vi "Test API Creates Report Folder.vi"(8 "error in (no error)":errorcluster, 11 "API Test in":refnum<class "API Test.lvclass">) -> (0 "error out":errorcluster, 3 "API Test out":refnum<class "API Test.lvclass">)   [LabVIEW 2020, in "LUnit Tests.lvlib" / "API Test.lvclass"]
uses:
  API Test.lvclass
  source/Framework/Execution API/Execution API.lvclass
  <vilib>/Astemes/LUnit/Test Case.lvclass
  C:/Program Files (x86)/National Instruments/LabVIEW 2020/vi.lib/Astemes/LUnit/Test Case.lvclass
  Test Dummys/Test Test Case/Test Test Case.lvclass
panel:
  out "file or folder exists?":bool
  out "appended path":path
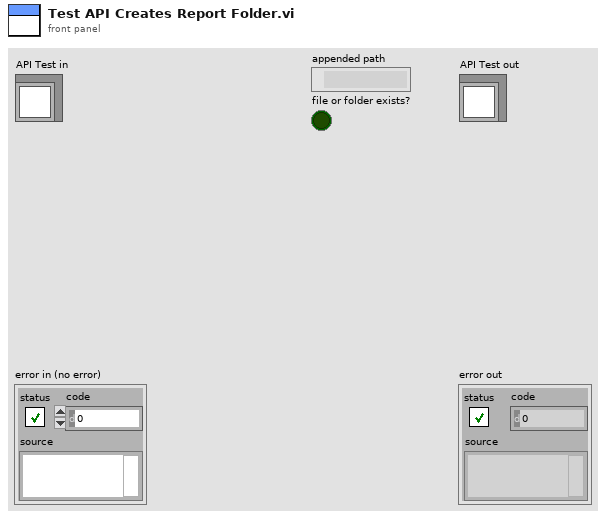
[diagram p1: front panel]
types:
  T1 = cluster{"Result Events":refnum<event-registration>, "Event Registration Refnum":refnum<event-registration>}
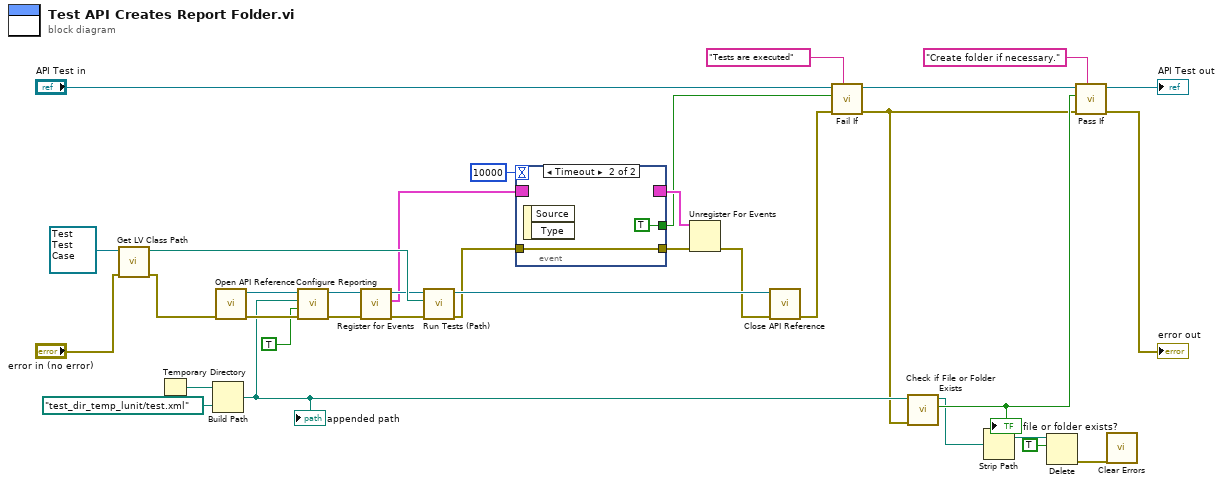
[diagram p0: block diagram]
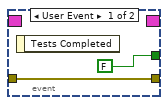
[diagram p2: hidden frame]
diagram:
  n1 = call <vilib>:"Get LV Class Path.vi"("error in (no error)"="error in (no error)", "object"=refnum<class "Test Test Case.lvclass"> refnum ("Test Test Case.lvclass")) -> ("error out"=w33:errorcluster, "class path"=w25:path)  [unwired: 8 in]
  n2 = Temporary Directory() -> (w24:path)
  n3 = Build Path(base path=w24, name or relative path=path "test_dir_temp_lunit/test.xml") -> (appended path=w21:path)
  "appended path" <- w21
  n4 = call "Open API Reference.vi"("error in (no error)"=w33) -> ("error out"=w27:errorcluster, "Execution API out"=w28:refnum<class "Execution API.lvclass">)  [unwired: 9 in]
  n5 = call "Configure Reporting.vi"("error in (no error)"=w27, "Autogenerate?"=TRUE, "Path"=w21, "Execution API In"=w28) -> ("error out"=w26:errorcluster, "Execution API Out"=w5:refnum<class "Execution API.lvclass">)  [unwired: 6 in]
  n6 = call "Register for Events.vi"("error in (no error)"=w26, "Execution API in"=w5) -> ("error out"=w6:errorcluster, "Event Registrations"=w3:T1, "Execution API out"=w4:refnum<class "Execution API.lvclass">)  [unwired: 7 in]
  n7 = call "Run Tests (Path).vi"("error in (no error)"=w6, "Project or Class Path"=w25, "Execution API In"=w4) -> ("error out"=w34:errorcluster, "Execution API Out"=w35:refnum<class "Execution API.lvclass">)  [unwired: 7 in]
  n8 = event shown="[1] Timeout" {
    selector: w3 -> [_ _]
    dyn-events: [_ _] -> w31
    timeout: 10000 -> [_ _]
    tunnel: [FALSE TRUE] -> w8
    tunnel: w34 -> [w36 w38]
    tunnel: [w36 w38] -> w30
    event User Event {
      n9 = event-data() -> ()  [unwired: 1 in, 1 out]
    }
    event Timeout {
      n10 = event-data() -> ()  [unwired: 1 in, 2 out]
    }
  }
  n11 = Unregister For Events(event registration refnum=w31, error in=w30) -> (error out=w32:errorcluster)
  n12 = call "Close API Reference.vi"("error in (no error)"=w32, "Execution API in"=w35) -> ("error out"=w13:errorcluster)  [unwired: 9 in]
  n13 = call <vilib>:"Fail If.vi"("Description"="Tests are executed", "error in (no error)"=w13, "Fail?"=w8, "LUnit Test Case In"="API Test in") -> ("error out"=w11:errorcluster, "LUnit Test Case Out"=w9:refnum<class "API Test.lvclass">)  [unwired: 6 in]
  n14 = call <vilib>:"Check if File or Folder Exists.vi"("error in (no error)"=w11, "path"=w21) -> ("file or folder exists?"=w18:bool, "dup path"=w17:path)  [unwired: 7 in, 1 out]
  "file or folder exists?" <- w18
  n15 = Strip Path(path=w17) -> (stripped path=w16:path)  [unwired: 1 out]
  n16 = Delete(path (use dialog)=w16, entire hierarchy (F)=TRUE) -> (error out=w1:errorcluster)  [unwired: 3 in, 2 out]
  n17 = call <vilib>:"Pass If.vi"("Description"="Create folder if necessary.", "error in (no error)"=w11, "Pass?"=w18, "LUnit Test Case In"=w9) -> ("error out"=→"error out":errorcluster, "LUnit Test Case Out"=→"API Test out":refnum<class "API Test.lvclass">)  [unwired: 6 in]
  n18 = call <vilib>:"Clear Errors.vi"("error in (no error)"=w1) -> ()  [unwired: 5 in, 2 out]
